vi "Add State(s) to Queue By BOOL(Array All).vi"(4 "False(\"\")":string[](array[string]), 6 "TRUE(\"\")":string[](array[string]), 8 "High Priority(FALSE)":bool, 10 "Bool":bool, 11 "State Queue(\"\")":string) -> (3 "State Queue Out":string)   [LabVIEW 2014, in "JKI State Machine++.lvlib"]
doc: "Depending on the High Priority and Bool input, this VI generates a concatenated state of TRUE/False and Remaining States. The High Priority input determines if the TRUE or False string concatenates before/after the remaining states. The Bool input determines whether TRUE or False string to be concatenated.\n\n<b>Inputs:</b>\n - <b>State Queue(\"\")</b>: The entire state queue is wired to this input.\n - <b>TRUE(\"\")</b>: State to insert when <b>Bool</b> is True.\n - <b>False(\"\")</b>: State to insert when <b>Bool</b> is False.\n - <b>Bool</b>: Flag for choosing State String connected to TRUE terminal or False terminal.\n - <b>High Priority(FALSE)</b>: If True, The state will be inserted to the top of the <b>State Queue(\"\")</b>. If False, It's appended to the tail.\n\n<b>Outputs:</b>\n - <b>State Queue Out</b>: Returns all the next states that should execute after the current state completes."
uses:
  JKI State Machine++.lvlib
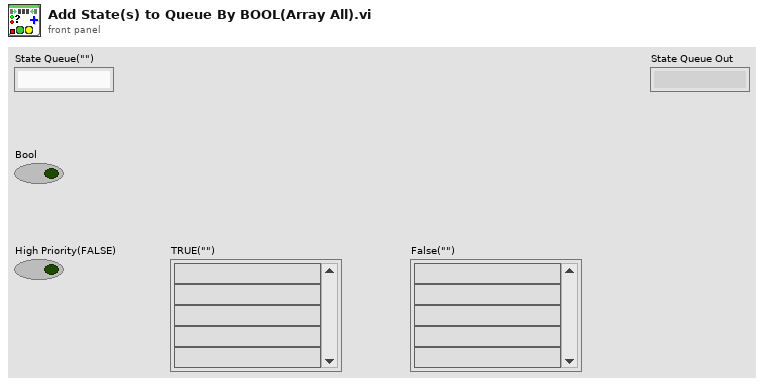
[diagram p1: front panel]
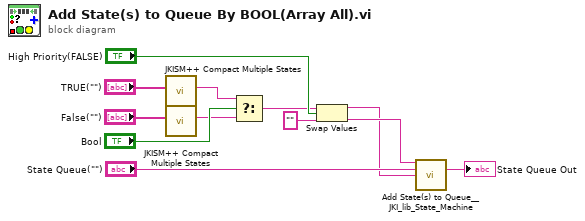
[diagram p0: block diagram]
diagram:
  n1 = call "JKISM++ Compact Multiple States.vi"("States in Lines"="TRUE(\"\")") -> ("States"=w2:string)  [unwired: 9 in]
  n2 = call "JKISM++ Compact Multiple States.vi"("States in Lines"="False(\"\")") -> ("States"=w1:string)  [unwired: 9 in]
  n3 = Select(t=w2, s="Bool", f=w1) -> (s? t:f=w6:string)
  n4 = Swap Values(12:w6, 13:"High Priority(FALSE)", 14:"") -> (1:w3:string, 3:w4:string)
  n5 = call <vilib>:"Add State(s) to Queue__JKI_lib_State_Machine.vi"("State(s) in Front (\"\")"=w4, "State(s) in (\"\")"="State Queue(\"\")", "State(s) at Back (\"\")"=w3) -> ("States Out"=→"State Queue Out":string)  [unwired: 12 in]
